vi "Initialize Frequency Task.vi"(0 "NI Force Task in":refnum<class "NI Force Task.lvclass">, 1 "Force Calibration Cluster":cluster{"Left":dbl, "Right":dbl}, 2 "TDMS File":refnum<k34>, 3 "EMG info":cluster{"Collect EMG?":bool, "EMG Rate":u16}, 4 "DAQ  Channels In":T1={"Force Transducer: Left"="Dev1/ai6", "Force Transducer: Right "="Dev1/ai8", "EMG: Left"="", "EMG: Right"="", "Potentiometer: Left"="", "Potentiometer: Right"=""}, 5 "error in (no error)":errorcluster, 9 "Task Info In":T2={"Number of Trials"=1, "Sampling Rate (Hz)"=200, "Trial Duration (s)"=10, "Adjusted MVC (N)"=5.0, "R Phase"=0, "L Phase"=0, "L Pattern"=1, "R Pattern"=1, "Time Between Trials (s)"=5, "Lissajous Speed"=200} {"Lissajous Speed" min=1 max=200; "Time Between Trials (s)" min=1 step=1; "R Pattern" min=1 max=20 step=1; "L Pattern" min=1 max=20 step=1; "L Phase" max=360 step=1; "R Phase" max=360 step=1; "Adjusted MVC (N)" min=1.0 step=1.0; "Trial Duration (s)" min=1 step=1; "Sampling Rate (Hz)" min=1 step=1; "Number of Trials" min=1 step=1}) -> (14 "NI Force Task out":refnum<class "NI Force Task.lvclass">, 19 "error out":errorcluster)   [LabVIEW 2020, in "NI Force Task.lvlib" / "NI Force Task.lvclass"]
uses:
  NI Force Task.lvclass
  Task info df.ctl
  NI Force Task.lvclass/NI Force Task.ctl
  <vilib>/DAQmx/create/channels.llb/DAQmx Create Channel (AI-Voltage-Basic).vi
  <vilib>/DAQmx/configure/timing.llb/DAQmx Timing (Sample Clock).vi
panel:
  out "error out 2":errorcluster
  # "Left Arm"
  # "Right Arm"
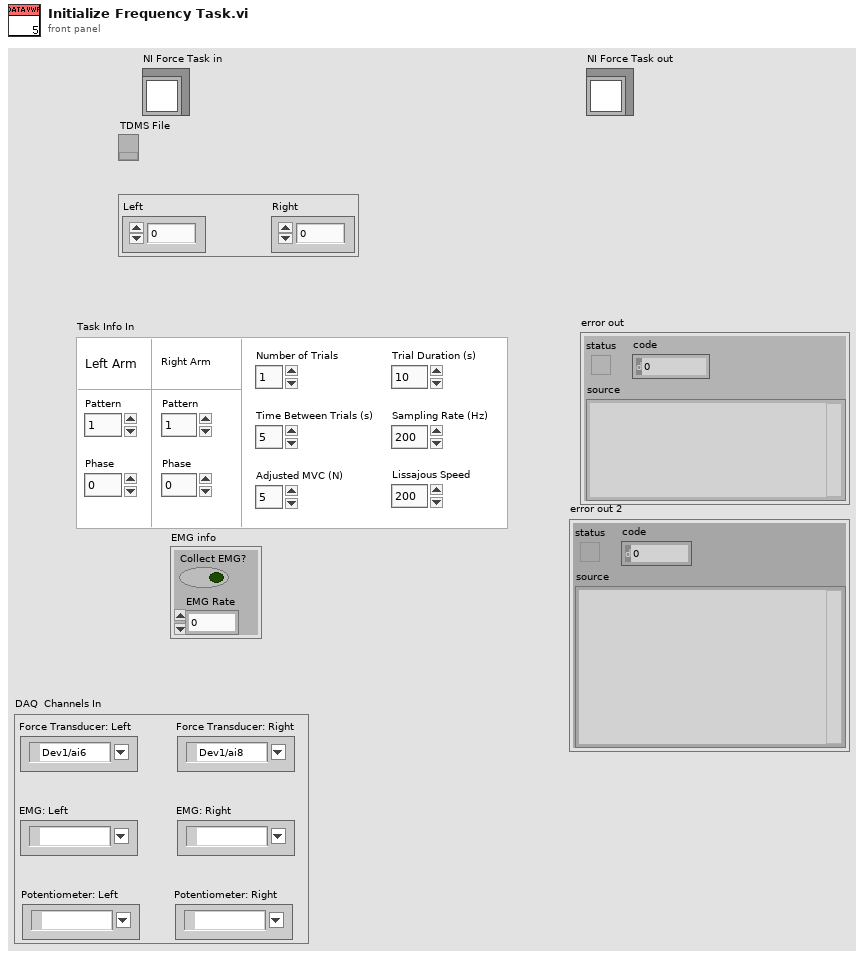
[diagram p1: front panel]
types:
  T1 = cluster{"Force Transducer: Left":tag, "Force Transducer: Right ":tag, "EMG: Left":tag, "EMG: Right":tag, "Potentiometer: Left":tag, "Potentiometer: Right":tag}
  T2 = typedef "Task info df.ctl" = cluster{"Number of Trials":u8, "Sampling Rate (Hz)":u16, "Trial Duration (s)":u8, "Adjusted MVC (N)":dbl, "R Phase":i32, "L Phase":i32, "L Pattern":u8, "R Pattern":u8, "Time Between Trials (s)":u8, "Lissajous Speed":u16}
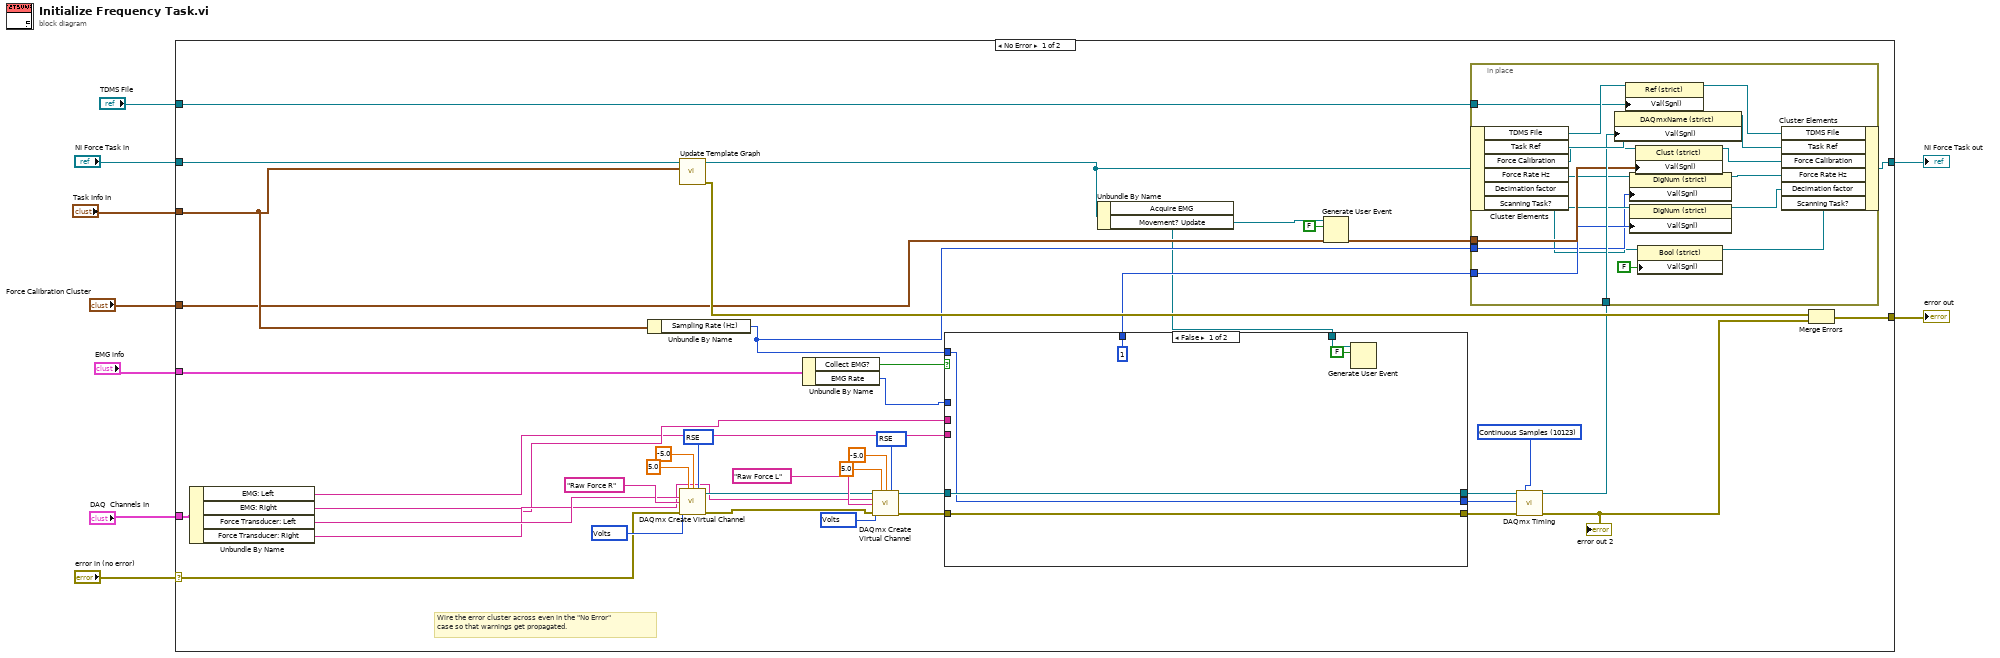
[diagram p0: block diagram]
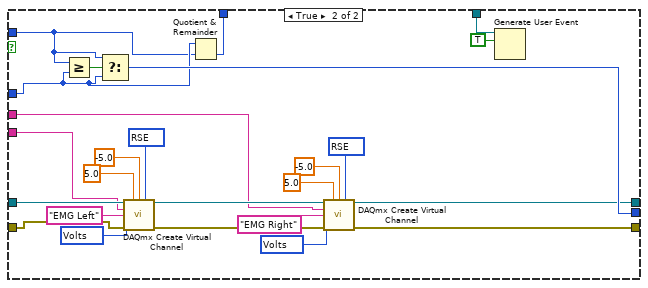
[diagram p2: hidden frame]
diagram:
  n1 = case shown="No Error" "error in (no error)" {
    selector: "error in (no error)" -> [w26 w102]
    tunnel: [w23 w102] -> w8
    tunnel: [w22 w101] -> w6
    tunnel: "NI Force Task in" -> [w51 w101]
    tunnel: "Task Info In" -> [w29 _]
    tunnel: "EMG info" -> [w50 _]
    tunnel: "DAQ  Channels In" -> [w48 _]
    tunnel: "Force Calibration Cluster" -> [w21 _]
    tunnel: "TDMS File" -> [w19 _]
    frame No Error {
      w27 = 10123 items=["Finite Samples"=10178, "Continuous Samples"=10123, "Hardware Timed Single Point"=12522] ("sample mode")
      w38 = 10348 items=["Volts"=10348, "From Custom Scale"=10065] ("units")
      w42 = 10083 items=["Default"=-1, "RSE"=10083, "NRSE"=10078, "Differential"=10106, "Pseudodifferential"=12529] ("input terminal configuration")
      w43 = 10348 items=["Volts"=10348, "From Custom Scale"=10065] ("units")
      w47 = 10083 items=["Default"=-1, "RSE"=10083, "NRSE"=10078, "Differential"=10106, "Pseudodifferential"=12529] ("input terminal configuration")
      # "Wire the error cluster across even in the \"No Error\"\ncase so that warnings get propagated."
      n2 = Unbundle By Name(w48) -> ("EMG: Left"=w16:tag, "EMG: Right"=w17:tag, "Force Transducer: Left"=w35:tag, "Force Transducer: Right"=w34:tag)
      n3 = Unbundle By Name(w29) -> ("Sampling Rate (Hz)"=w14:u16)
      n4 = call "Update Template Graph.vi"("Task Info In"=w29, "NI Force Task in"=w51) -> ("error out"=w25:errorcluster, "NI Force Task out"=w13:refnum<class "NI Force Task.lvclass">)  [unwired: 8 in]
      n5 = call-poly <vilib>:"DAQmx Create Virtual Channel.vi"("maximum value"=5.0, "minimum value"=-5.0, "input terminal configuration"=w47, "physical channels"=w35, "name to assign"="Raw Force R", "units"=w43, "error in"=w26) -> ("task out"=w37:refnum<k21>, "error out"=w36:errorcluster)  [unwired: 7 in]
      n6 = Unbundle By Name(w50) -> ("Collect EMG?"=w49:bool, "EMG Rate"=w28:u16)
      n7 = call-poly <vilib>:"DAQmx Create Virtual Channel.vi"("task in"=w37, "maximum value"=5.0, "minimum value"=-5.0, "input terminal configuration"=w42, "physical channels"=w34, "name to assign"="Raw Force L", "units"=w38, "error in"=w36) -> ("task out"=w33:refnum<k21>, "error out"=w32:errorcluster)  [unwired: 6 in]
      n8 = Unbundle By Name(w13) -> ("Acquire EMG"=w12:refnum<user-event>, "Movement? Update"=w11:refnum<user-event>)
      n9 = case shown="False" w49 {
        tunnel: w33 -> [w57 w72]
        tunnel: [w57 w64] -> w31
        tunnel: [w56 w63] -> w30
        tunnel: w32 -> [w56 w71]
        tunnel: w14 -> [w55 w61]
        tunnel: w28 -> [_ w62]
        tunnel: [w55 w81] -> w18
        tunnel: w17 -> [_ w66]
        tunnel: w16 -> [_ w65]
        tunnel: [u16 1 w60] -> w15
        tunnel: w12 -> [w53 w59]
        frame False {
          n10 = Generate User Event(user event=w53, event data cluster=FALSE ("event data")) -> ()  [unwired: 2 in, 2 out]
        }
        frame True {
          w73 = 10348 items=["Volts"=10348, "From Custom Scale"=10065] ("units")
          w76 = 10083 items=["Default"=-1, "RSE"=10083, "NRSE"=10078, "Differential"=10106, "Pseudodifferential"=12529] ("input terminal configuration")
          w77 = 10348 items=["Volts"=10348, "From Custom Scale"=10065] ("units")
          w80 = 10083 items=["Default"=-1, "RSE"=10083, "NRSE"=10078, "Differential"=10106, "Pseudodifferential"=12529] ("input terminal configuration")
          n11 = Greater Or Equal?(x=w61, y=w62) -> (x >= y?=w82:bool)
          n12 = Select(t=w61, s=w82, f=w62) -> (s? t:f=w81:u16)
          n13 = call-poly <vilib>:"DAQmx Create Virtual Channel.vi"("task in"=w72, "maximum value"=5.0, "minimum value"=-5.0, "input terminal configuration"=w80, "physical channels"=w65, "name to assign"="EMG Left", "units"=w77, "error in"=w71) -> ("task out"=w70:refnum<k21>, "error out"=w69:errorcluster)  [unwired: 6 in]
          n14 = Quotient & Remainder(x=w62, y=w61) -> (floor(x/y)=w60:u16)  [unwired: 1 out]
          n15 = call-poly <vilib>:"DAQmx Create Virtual Channel.vi"("task in"=w70, "maximum value"=5.0, "minimum value"=-5.0, "input terminal configuration"=w76, "physical channels"=w66, "name to assign"="EMG Right", "units"=w73, "error in"=w69) -> ("task out"=w64:refnum<k21>, "error out"=w63:errorcluster)  [unwired: 6 in]
          n16 = Generate User Event(user event=w59, event data cluster=TRUE ("event data")) -> ()  [unwired: 2 in, 2 out]
        }
      }
      n17 = Generate User Event(user event=w11, event data cluster=FALSE ("event data")) -> ()  [unwired: 2 in, 2 out]
      n18 = call-poly <vilib>:"DAQmx Timing.vi"("task/channels in"=w31, "sample mode"=w27, "rate"=w18, "error in"=w30) -> ("task out"=w20:refnum<k21>, "error out"=w24:errorcluster)  [unwired: 10 in]
      "error out 2" <- w24
      n19 = in-place {
        in-place-border: w21 -> [w92]
        in-place-border: w20 -> [w98]
        in-place-border: w19 -> [w97]
        in-place-border: w15 -> [w87]
        in-place-border: w14 -> [w86]
        n20 = in-place-cluster #1(w13) -> ("TDMS File"=w100:refnum<vi>, "Task Ref"=w99:refnum<vi>, "Force Calibration"=w94:refnum<vi>, "Force Rate Hz"=w91:refnum<vi>, "Decimation factor"=w89:refnum<vi>, "Scanning Task?"=w85:refnum<vi>)
        n21 = property class="DAQmxName (strict)"(reference=w99, "Val(Sgnl)"=w98) -> (reference out=w95:refnum<vi>)  [unwired: 1 in, 1 out]
        n22 = property class="Ref (strict)"(reference=w100, "Val(Sgnl)"=w97) -> (reference out=w96:refnum<vi>)  [unwired: 1 in, 1 out]
        n23 = property class="DigNum (strict)"(reference=w91, "Val(Sgnl)"=w86) -> (reference out=w90:refnum<vi>)  [unwired: 1 in, 1 out]
        n24 = property class="DigNum (strict)"(reference=w89, "Val(Sgnl)"=w87) -> (reference out=w88:refnum<vi>)  [unwired: 1 in, 1 out]
        n25 = property class="Clust (strict)"(reference=w94, "Val(Sgnl)"=w92) -> (reference out=w93:refnum<vi>)  [unwired: 1 in, 1 out]
        n26 = property class="Bool (strict)"(reference=w85, "Val(Sgnl)"=FALSE ("Value (Signaling)")) -> (reference out=w84:refnum<vi>)  [unwired: 1 in, 1 out]
        n27 = in-place-cluster #1("TDMS File"=w96, "Task Ref"=w95, "Force Calibration"=w93, "Force Rate Hz"=w90, "Decimation factor"=w88, "Scanning Task?"=w84) -> (w22:refnum<class "NI Force Task.lvclass">)
      }
      n28 = Merge Errors(w25, w24) -> (w23:errorcluster)
    }
    frame Error {
    }
  }
  "error out" <- w8
  "NI Force Task out" <- w6
